vi "RemoveChannel Value Change.vi"(10 "channel":i32, 11 "References":T1) -> (0 "error out":errorcluster)   [LabVIEW 2015, in "TDMS datalogger editor node.lvclass"]
uses:
  TDMS datalogger editor node.lvclass
  <vilib>/NI/DCAF/Tag Editor Core/Table API/Table Manager/object ref.ctl
  <vilib>/NI/DCAF/Tag Editor Core/Configuration Editor/Classes/Engine Parent/Engine Parent Editor Node.lvclass
  <vilib>/NI/DCAF/Tag Editor Core/Configuration Editor/Classes/Module editor node/module editor node.lvclass
  TDMS datalogger editor node.lvclass/TDMS datalogger editor node.ctl
  <vilib>/NI/Configuration Framework/serializable configuration/NISE_CEF_serializable configuration.lvclass/NISE_CEF_serializable configuration.ctl
  <vilib>/Utility/LVClass/Get LV Class Name.vi
  <vilib>/NI/Configuration Framework/error generator/NISE_error generator.vi
  module/configuration/TDMS datalogger configuration.lvclass
  <vilib>/NI/Module Execution Interface/Engine Configuration/engine configuration.lvclass
  <vilib>/NI/Configuration Framework/serializable configuration/NISE_CEF_serializable configuration.lvclass
  <vilib>/NI/DCAF/Tag Editor Core/Table API/Table Manager/Table Manager.lvclass
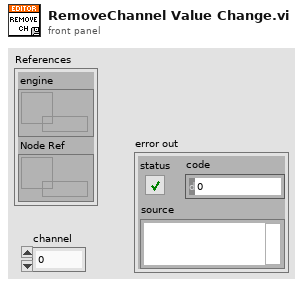
[diagram p1: front panel]
types:
  T1 = typedef "Table Manager.lvlib/Table Manager.lvclass/object ref.ctl" = cluster{"engine":refnum<data-value>, "Node Ref":refnum<data-value>}
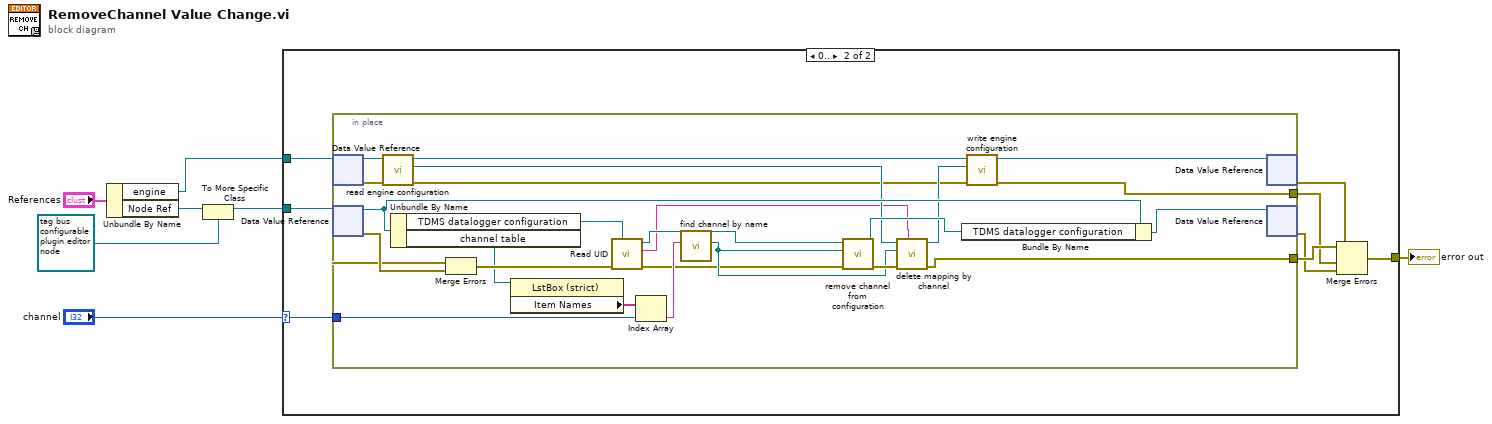
[diagram p0: block diagram]
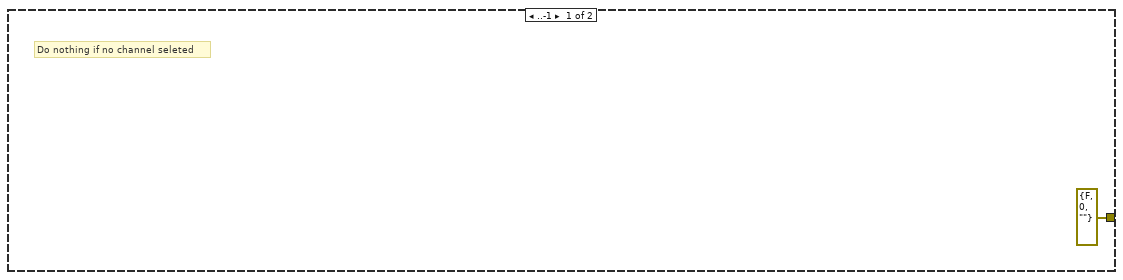
[diagram p2: hidden frame]
diagram:
  n1 = Unbundle By Name("References") -> ("engine"=w3:refnum<data-value>, "Node Ref"=w6:refnum<data-value>)
  n2 = To More Specific Class(target class=refnum<data-value> refnum ("data value reference"), reference=w6) -> (specific class reference=w4:refnum<data-value>)  [unwired: 1 in, 1 out]
  n3 = case shown="0.." "channel" {
    selector: "channel" -> [_ w10]
    tunnel: [errorcluster {"status"=FALSE, "code"=0, "source"=""} ("error IO") w12] -> w1
    tunnel: w4 -> [_ w11]
    tunnel: w3 -> [_ w9]
    frame ..-1 {
      # "Do nothing if no channel seleted"
    }
    frame 0.. {
      n4 = in-place {
        in-place-border: [w25] -> w16
        in-place-border: [w35] -> w15
        in-place-border: w10 -> [w27]
        n5 = in-place-dvr #1(w9) -> (w37:refnum<class "Engine Parent Editor Node.lvclass">, w38:errorcluster)
        n6 = in-place-dvr #2(w11) -> (w34:refnum<class "TDMS datalogger editor node.lvclass">, w40:errorcluster)
        n7 = call <vilib>:"read engine configuration.vi"("error in"=w38, "Engine Parent Editor Node in"=w37) -> ("error out"=w23:errorcluster, "engine configuration"=w26:refnum<class "engine configuration.lvclass">, "Engine Parent Editor Node out"=w36:refnum<class "Engine Parent Editor Node.lvclass">)  [unwired: 7 in]
        n8 = Unbundle By Name(w34) -> ("TDMS datalogger configuration"=w21:refnum<class "TDMS datalogger configuration.lvclass">, "channel table"=w18:refnum<vi>)
        n9 = Merge Errors(w23, w40) -> (w28:errorcluster)
        n10 = property class="LstBox (strict)"(reference=w18) -> ("Item Names"=w17:string[])  [unwired: 1 in, 2 out]
        n11 = call <vilib>:"Read UID.vi"("error in"=w28, "configuration in"=w21) -> ("error out"=w22:errorcluster, "instance id"=w19:string, "configuration out"=w20:refnum<class "TDMS datalogger configuration.lvclass">)  [unwired: 7 in]
        n12 = Index Array(array=w17, index=w27) -> (element=w31:string)
        n13 = call "find channel by name.vi"("channel name"=w31, "TDMS datalogger configuration in"=w20) -> ("channel"=w30:refnum<class "TBM channel.lvclass">, "TDMS datalogger configuration out"=w32:refnum<class "TDMS datalogger configuration.lvclass">)  [unwired: 8 in]
        n14 = call "remove channel from configuration.vi"("error in"=w22, "TBM channel in"=w30, "TDMS datalogger configuration in"=w32) -> ("error out"=w33:errorcluster, "TDMS datalogger configuration out"=w29:refnum<class "TDMS datalogger configuration.lvclass">)  [unwired: 7 in]
        n15 = call <vilib>:"delete mapping by channel.vi"("owner ID"=w19, "error in"=w33, "channel"=w30, "engine configuration in"=w26) -> ("error out"=w25:errorcluster, "engine configuration out"=w24:refnum<class "engine configuration.lvclass">)  [unwired: 6 in]
        n16 = Bundle By Name(cluster=w34, "TDMS datalogger configuration"=w29) -> (w41:refnum<class "TDMS datalogger editor node.lvclass">)
        n17 = call <vilib>:"write engine configuration.vi"("error in"=w23, "engine configuration"=w24, "Engine Parent Editor Node in"=w36) -> ("error out"=w35:errorcluster, "Engine Parent Editor Node out"=w39:refnum<class "Engine Parent Editor Node.lvclass">)  [unwired: 7 in]
        n18 = in-place-dvr #1(w39) -> (w14:errorcluster)  [unwired: 1 out]
        n19 = in-place-dvr #2(w41) -> (w13:errorcluster)  [unwired: 1 out]
      }
      n20 = Merge Errors(w16, w14, w15, w13) -> (w12:errorcluster)
    }
  }
  "error out" <- w1
